vi "Double_GeneralGearShift_WithDeadTime (3).vi"(6 "error In":errorcluster, 7 "ShifterRef":T1={"DevStatus"={"status"=FALSE, "code"=0, "source"=""}, "Pneumatics Control Module"=0, "Forward Solenoid Channel"=enum."Invalid", "Reverse Solenoid Channel"=enum."Invalid"}, 8 "Shift Control":bool, 9 "Shift Value":T3, 10 "Right":dbl, 11 "Left":dbl) -> (0 "error out":errorcluster, 1 "Shifting":bool, 2 "Right Output":dbl, 3 "Left Output":dbl)   [LabVIEW 2016]
uses:
  <vilib>/Rock Robotics/WPI/Solenoid/WPI_SolenoidValue.ctl
  <vilib>/Rock Robotics/WPI/Solenoid/WPI_SolenoidDevRef.ctl
  <vilib>/Rock Robotics/WPI/Solenoid/WPI_SolenoidChannel.ctl
  <vilib>/Rock Robotics/WPI/ThirdParty/CanMotor/TalonSRX/WPI_CANTalonSRX_BrakeOverride.ctl
  <vilib>/Rock Robotics/WPI/Solenoid/WPI_SolenoidSetEnum.vi
panel:
  out "Right Starting Point":dbl
  out "Left Starting Point":dbl
  out "TempTimeVal":u32
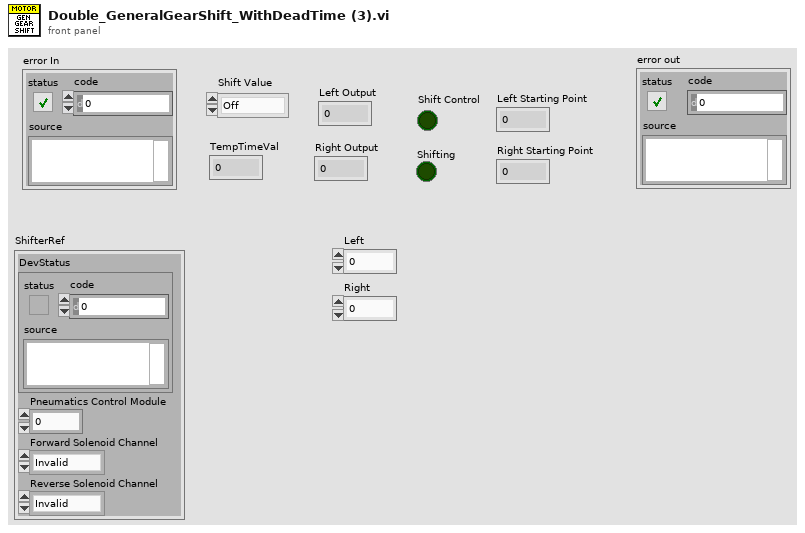
[diagram p1: front panel]
types:
  T1 = typedef "WPI_SolenoidDevRef.ctl" = cluster{"DevStatus":errorcluster, "Pneumatics Control Module":u8, "Forward Solenoid Channel":T2, "Reverse Solenoid Channel":T2}
  T2 = typedef "WPI_SolenoidChannel.ctl" = enum8{"Solenoid 0", "Solenoid 1", "Solenoid 2", "Solenoid 3", "Solenoid 4", "Solenoid 5", "Solenoid 6", "Solenoid 7", "Invalid"}
  T3 = typedef "WPI_SolenoidValue.ctl" = enum16{"Off", "On", "Forward", "Reverse"}
  T4 = typedef "WPI_MotorControlDeviceRef.ctl" = cluster{"DeviceStatus":errorcluster, "Type":T5, "PWM":cluster{"PWM Channel":T6, "DeadBand":T7}, "CAN":cluster{"Device Number":u8, "SetOutput VI Ref":variant, "GetOutput VI Ref":variant, "Enable VI Ref":variant, "Disable VI Ref":variant, "Data":variant}, "Invert":bool}
  T5 = typedef "WPI_MotorControlType.ctl" = enum16{"PWM", "CAN"}
  T6 = typedef "FPGA_DIOPWMChannel.ctl" = enum8{"PWM 0", "PWM 1", "PWM 2", "PWM 3", "PWM 4", "PWM 5", "PWM 6", "PWM 7", "PWM 8", "PWM 9", "PWM MXP 0", "PWM MXP 1", "PWM MXP 2", "PWM MXP 3", "PWM MXP 4", "PWM MXP 5", "PWM MXP 6", "PWM MXP 7", "PWM MXP 8", "PWM MXP 9", "Invalid"}
  T7 = typedef "WPI_PWMDeadband.ctl" = cluster{"Name":string, "maxPositivePwm":i32, "minPositivePwm":i32, "centerPwm":i32, "maxNegativePwm":i32, "minNegativePwm":i32, "angularRange":u16}
  T8 = typedef "WPI_CANTalonSRX_BrakeOverride.ctl" = enum8{"No Override", "Override to Coast", "Override to Brake"}
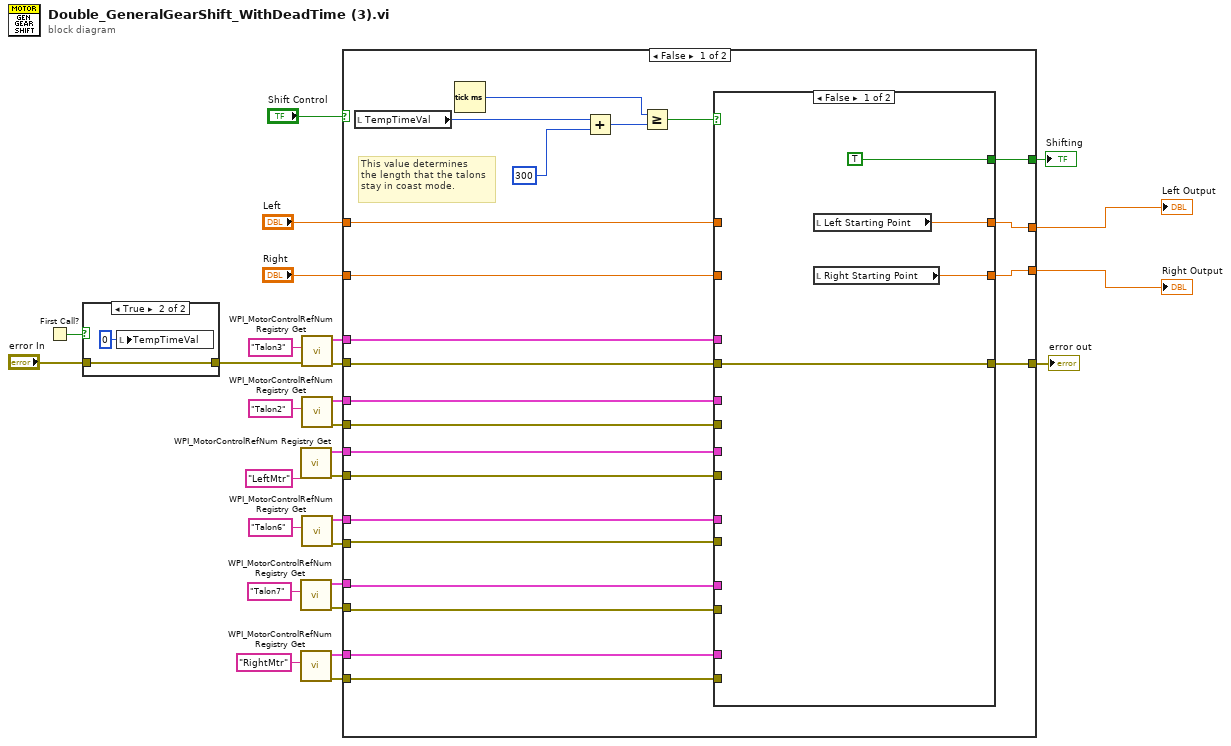
[diagram p0: block diagram]
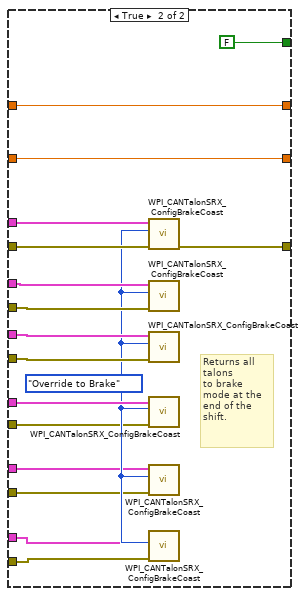
[diagram p3: hidden frame]
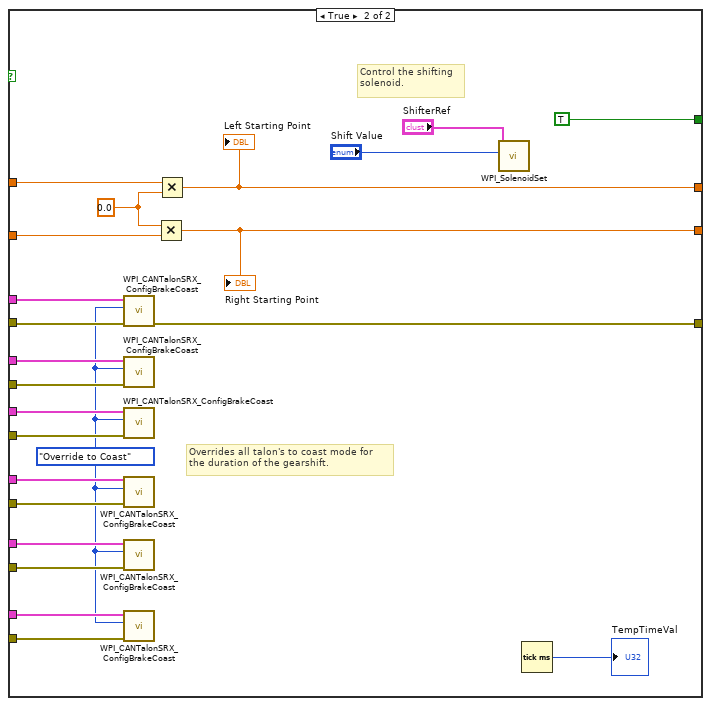
[diagram p4: hidden frame]
diagram:
  n1 = First Call?() -> (First Call?: T/F=w23:bool)
  n2 = case shown="True" w23 {
    tunnel: [w29 w30] -> w19
    tunnel: "error In" -> [w29 w30]
    frame False {
    }
    frame True {
      n3 = local write "TempTimeVal"(u32 0 ("TempTimeVal")) -> ()
    }
  }
  n4 = call <vilib>:"WPI_MotorControlRefNum Registry Get.vi"("refnum name"="LeftMtr") -> ("error out"=w13:errorcluster, "MotorControlDevRef"=w14:T4)  [unwired: 9 in]
  n5 = call <vilib>:"WPI_MotorControlRefNum Registry Get.vi"("refnum name"="Talon7") -> ("error out"=w9:errorcluster, "MotorControlDevRef"=w10:T4)  [unwired: 9 in]
  n6 = call <vilib>:"WPI_MotorControlRefNum Registry Get.vi"("refnum name"="RightMtr") -> ("error out"=w7:errorcluster, "MotorControlDevRef"=w8:T4)  [unwired: 9 in]
  n7 = call <vilib>:"WPI_MotorControlRefNum Registry Get.vi"("error in (no error)"=w19, "refnum name"="Talon3") -> ("error out"=w18:errorcluster, "MotorControlDevRef"=w17:T4)  [unwired: 8 in]
  n8 = call <vilib>:"WPI_MotorControlRefNum Registry Get.vi"("refnum name"="Talon2") -> ("error out"=w15:errorcluster, "MotorControlDevRef"=w16:T4)  [unwired: 9 in]
  n9 = call <vilib>:"WPI_MotorControlRefNum Registry Get.vi"("refnum name"="Talon6") -> ("error out"=w11:errorcluster, "MotorControlDevRef"=w12:T4)  [unwired: 9 in]
  n10 = case shown="False" "Shift Control" {
    tunnel: [w54 w92] -> w28
    tunnel: [w53 w91] -> w27
    tunnel: "Right" -> [w52 w96]
    tunnel: "Left" -> [w51 w97]
    tunnel: w18 -> [w47 w95]
    tunnel: [w44 w94] -> w21
    tunnel: [w43 TRUE] -> w20
    tunnel: w17 -> [w42 w87]
    tunnel: w16 -> [w41 w86]
    tunnel: w15 -> [w40 w85]
    tunnel: w14 -> [w39 w84]
    tunnel: w13 -> [w38 w83]
    tunnel: w12 -> [w37 w82]
    tunnel: w11 -> [w36 w81]
    tunnel: w10 -> [w35 w80]
    tunnel: w9 -> [w34 w79]
    tunnel: w8 -> [w33 w78]
    tunnel: w7 -> [w32 w77]
    frame False {
      # "This value determines\nthe length that the talons\nstay in coast mode."
      n11 = local read "TempTimeVal"() -> (w46:u32)
      n12 = Tick Count (ms)() -> (millisecond timer value=w49:u32)
      n13 = Add(x=w46, y=300) -> (x+y=w48:u32)
      n14 = Greater Or Equal?(x=w49, y=w48) -> (x >= y?=w50:bool)
      n15 = case shown="False" w50 {
        tunnel: [w56 w74] -> w54
        tunnel: [w57 w75] -> w53
        tunnel: w52 -> [_ w75]
        tunnel: w51 -> [_ w74]
        tunnel: w47 -> [w58 w73]
        tunnel: [w58 w72] -> w44
        tunnel: [TRUE FALSE] -> w43
        tunnel: w42 -> [_ w70]
        tunnel: w41 -> [_ w69]
        tunnel: w40 -> [_ w68]
        tunnel: w39 -> [_ w67]
        tunnel: w38 -> [_ w66]
        tunnel: w37 -> [_ w65]
        tunnel: w36 -> [_ w63]
        tunnel: w35 -> [_ w62]
        tunnel: w34 -> [_ w61]
        tunnel: w33 -> [_ w60]
        tunnel: w32 -> [_ w59]
        frame False {
          n16 = local read "Left Starting Point"() -> (w56:dbl)
          n17 = local read "Right Starting Point"() -> (w57:dbl)
        }
        frame True {
          w64 = WPI_CANTalonSRX_BrakeOverride."Override to Brake" ("Brake / Coast Mode")
          # "Returns all talons\nto brake mode at the\nend of the shift."
          n18 = call <vilib>:"WPI_CANTalonSRX_ConfigBrakeCoast.vi"("error in (no error)"=w73, "Brake / Coast Mode"=w64, "CAN Talon SRX Ref"=w70) -> ("error out"=w72:errorcluster)  [unwired: 7 in, 1 out]
          n19 = call <vilib>:"WPI_CANTalonSRX_ConfigBrakeCoast.vi"("error in (no error)"=w68, "Brake / Coast Mode"=w64, "CAN Talon SRX Ref"=w69) -> ()  [unwired: 7 in, 2 out]
          n20 = call <vilib>:"WPI_CANTalonSRX_ConfigBrakeCoast.vi"("error in (no error)"=w66, "Brake / Coast Mode"=w64, "CAN Talon SRX Ref"=w67) -> ()  [unwired: 7 in, 2 out]
          n21 = call <vilib>:"WPI_CANTalonSRX_ConfigBrakeCoast.vi"("error in (no error)"=w63, "Brake / Coast Mode"=w64, "CAN Talon SRX Ref"=w65) -> ()  [unwired: 7 in, 2 out]
          n22 = call <vilib>:"WPI_CANTalonSRX_ConfigBrakeCoast.vi"("error in (no error)"=w61, "Brake / Coast Mode"=w64, "CAN Talon SRX Ref"=w62) -> ()  [unwired: 7 in, 2 out]
          n23 = call <vilib>:"WPI_CANTalonSRX_ConfigBrakeCoast.vi"("error in (no error)"=w59, "Brake / Coast Mode"=w64, "CAN Talon SRX Ref"=w60) -> ()  [unwired: 7 in, 2 out]
        }
      }
    }
    frame True {
      w76 = WPI_CANTalonSRX_BrakeOverride."Override to Coast" ("Brake / Coast Mode")
      w93 = 0.0
      # "Control the shifting\nsolenoid."
      # "Overrides all talon's to coast mode for \nthe duration of the gearshift."
      n24 = call <vilib>:"WPI_CANTalonSRX_ConfigBrakeCoast.vi"("error in (no error)"=w95, "Brake / Coast Mode"=w76, "CAN Talon SRX Ref"=w87) -> ("error out"=w94:errorcluster)  [unwired: 7 in, 1 out]
      n25 = call <vilib>:"WPI_CANTalonSRX_ConfigBrakeCoast.vi"("error in (no error)"=w85, "Brake / Coast Mode"=w76, "CAN Talon SRX Ref"=w86) -> ()  [unwired: 7 in, 2 out]
      n26 = call <vilib>:"WPI_CANTalonSRX_ConfigBrakeCoast.vi"("error in (no error)"=w83, "Brake / Coast Mode"=w76, "CAN Talon SRX Ref"=w84) -> ()  [unwired: 7 in, 2 out]
      n27 = call <vilib>:"WPI_CANTalonSRX_ConfigBrakeCoast.vi"("error in (no error)"=w81, "Brake / Coast Mode"=w76, "CAN Talon SRX Ref"=w82) -> ()  [unwired: 7 in, 2 out]
      n28 = call <vilib>:"WPI_CANTalonSRX_ConfigBrakeCoast.vi"("error in (no error)"=w79, "Brake / Coast Mode"=w76, "CAN Talon SRX Ref"=w80) -> ()  [unwired: 7 in, 2 out]
      n29 = call <vilib>:"WPI_CANTalonSRX_ConfigBrakeCoast.vi"("error in (no error)"=w77, "Brake / Coast Mode"=w76, "CAN Talon SRX Ref"=w78) -> ()  [unwired: 7 in, 2 out]
      n30 = Multiply(x=w93, y=w96) -> (x*y=w91:dbl)
      "Right Starting Point" <- w91
      n31 = Multiply(x=w97, y=w93) -> (x*y=w92:dbl)
      "Left Starting Point" <- w92
      n32 = call-poly <vilib>:"WPI_SolenoidSet.vi"("Value"="Shift Value", "SolenoidDevRef"="ShifterRef") -> ()  [unwired: 8 in, 2 out]
      n33 = Tick Count (ms)() -> (millisecond timer value=→"TempTimeVal":u32)
    }
  }
  "Left Output" <- w28
  "Right Output" <- w27
  "error out" <- w21
  "Shifting" <- w20
